vi "Get Path Regex.vi"(8 "error in (no error)":errorcluster, 11 "TestCSRFController in":refnum<class "TestCSRFController.lvclass">) -> (0 "error out":errorcluster, 2 "Path Regex":string, 3 "TestCSRFController out":refnum<class "TestCSRFController.lvclass">)   [LabVIEW 2020, in "TestCSRFController.lvclass"]
uses:
  TestCSRFController.lvclass
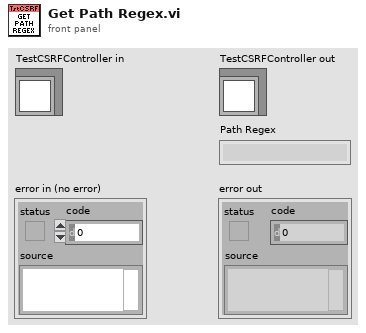
[diagram p1: front panel]
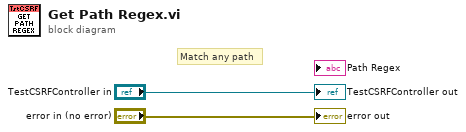
[diagram p0: block diagram]
diagram:
  # "Match any path"
  "error out" <- "error in (no error)"
  "TestCSRFController out" <- "TestCSRFController in"
